vi "WPI_ErrDMAAlreadyStarted.vi"() -> (0 "error out":errorcluster)   [LabVIEW 2017]
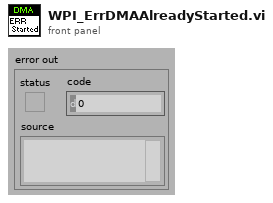
[diagram p1: front panel]
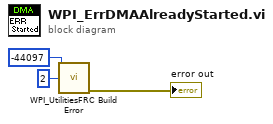
[diagram p0: block diagram]
diagram:
  n1 = call <vilib>:"WPI_UtilitiesFRC Build Error.vi"("error code"=-44097 ("code"), "chain levels to remove (1)"=2) -> ("error out"=→"error out":errorcluster)  [unwired: 3 in, 10 out]
